vi "Is section control.vi"(8 "error in":errorcluster, 11 "control reference in":refnum<vi>) -> (0 "error out":errorcluster, 1 "First Section":bool, 2 "Section":bool, 3 "control reference out":refnum<vi>)   [LabVIEW 2020, in "verticalDistribution.lvlib"]
uses:
  <vilib>/Utility/vertDist/verticalDistribution.lvlib
  <vilib>/Utility/vertDist/FirstSectionLabel.ctl
  <vilib>/Utility/vertDist/SectionLabel.ctl
panel:
  out "First Section":T1="Sample First Section"
  out "General Section":T2="Sample Section"
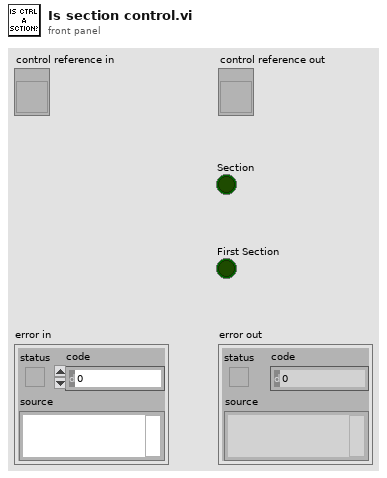
[diagram p1: front panel]
types:
  T1 = typedef "verticalDistribution.lvlib/FirstSectionLabel.ctl" = string
  T2 = typedef "verticalDistribution.lvlib/SectionLabel.ctl" = string
  T3 = enum32{"not a typedef", "typedef", "strict typedef", "class private data"}
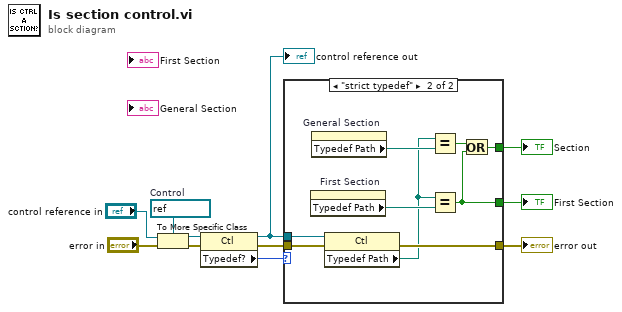
[diagram p0: block diagram]
diagram:
  w7 = refnum<vi> refnum  # Control
  n1 = To More Specific Class(target class=w7, reference="control reference in", error in="error in") -> (specific class reference=w6:refnum<vi>, error out=w10:errorcluster)
  n2 = property class="Ctl"(reference=w6, error in=w10) -> (reference out=w4:refnum<vi>, error out=w9:errorcluster, "Typedef?"=w5:T3)
  "control reference out" <- w4
  n3 = case shown="\"strict typedef\"" w5 {
    tunnel: w4 -> [_ w19]
    tunnel: w9 -> [w12 w21]
    tunnel: [w12 w20] -> w8
    tunnel: [_ w14] -> w2
    tunnel: [_ w13] -> w1
    frame Default {
    }
    frame "strict typedef" {
      n4 = property on="First Section" class="Str (strict)"() -> ("Typedef Path"=w17:path)  [unwired: 2 in, 2 out]
      n5 = property on="General Section" class="Str (strict)"() -> ("Typedef Path"=w18:path)  [unwired: 2 in, 2 out]
      n6 = property class="Ctl"(reference=w19, error in=w21) -> (error out=w20:errorcluster, "Typedef Path"=w16:path)  [unwired: 1 out]
      n7 = Equal?(x=w16, y=w18) -> (x = y?=w15:bool)
      n8 = Equal?(x=w16, y=w17) -> (x = y?=w13:bool)
      n9 = Or(x=w15, y=w13) -> (x .or. y?=w14:bool)
    }
  }
  "error out" <- w8
  "Section" <- w2
  "First Section" <- w1
